vi "ex_EscUnprintChars.vi"(1 "input":string) -> (0 "output":string)   [LabVIEW 2017]
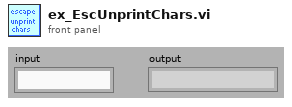
[diagram p1: front panel]
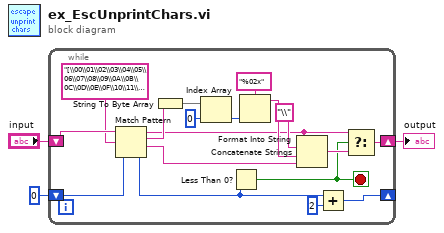
[diagram p0: block diagram]
diagram:
  n1 = while {
    shift-left: 0 -> [w20]
    shift-right: [w19] -> _
    shift-left: "input" -> [w21]
    shift-right: [w6] -> w2
    stop <- w4 stop-if-true
    n2 = Match Pattern(string=w21, regular expression="[\\00\\01\\02\\03\\04\\05\\06\\07\\08\\09\\0A\\0B\\0C\\0D\\0E\\0F\\10\\11\\12\\13\\14\\15\\16\\17\\18\\19\\1A\\1B\\1C\\1D\\1E\\1F]", offset (0)=w20) -> (before substring=w8:string, match substring=w16:string, after substring=w17:string, offset past match=w9:i32)
    n3 = String To Byte Array(string=w16) -> (unsigned byte array=w15:u8[])
    n4 = Index Array(array=w15, index=0) -> (element=w13:u8)
    n5 = Less Than 0?(x=w9) -> (x < 0?=w4:bool)
    n6 = Format Into String(format string="%02x", w13) -> (resulting string=w11:string)  [unwired: 2 in, 1 out]
    n7 = Concatenate Strings(w8, "\\", w11, w17) -> (w7:string)
    n8 = Add(x=w9, y=2 ("offset past match")) -> (x+y=w19:i32)
    n9 = Select(t=w8, s=w4, f=w7) -> (s? t:f=w6:string)
  }
  "output" <- w2
